vi "main.vi"() -> ()   [LabVIEW 2015]
doc: "Reading data from an ini file. Sorting using the array function. Writing sorted data to an ini file."
panel:
  out "errors when writing the ini file":errorcluster
  in  "Sorted and recorded file":path
  out "errors when reading the ini file":errorcluster
  in  "Source file":path
  in  "cluster structure":T1
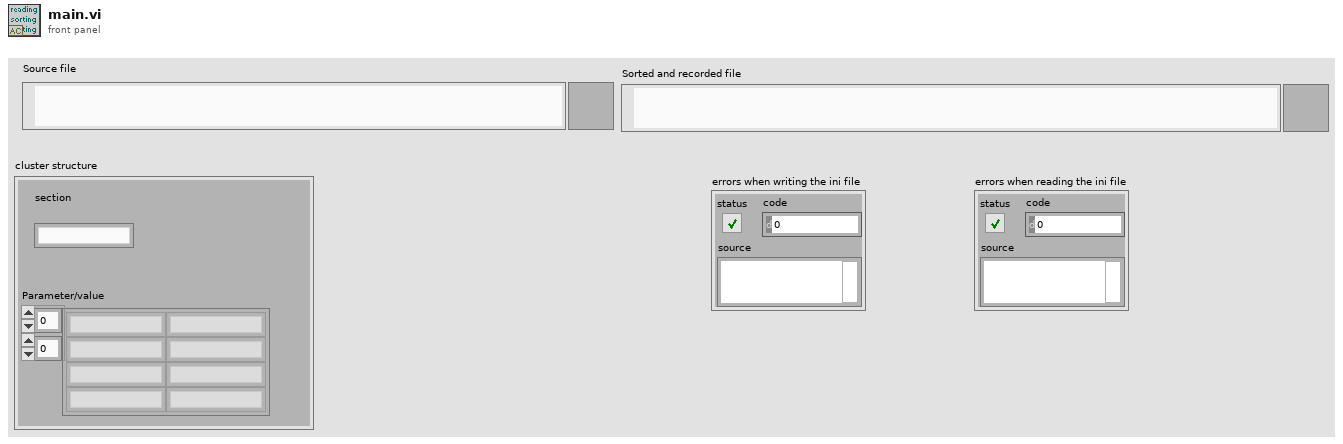
[diagram p1: front panel]
types:
  T1 = cluster{"section\n":string, "Parameter/value":string[][]}
  T2 = cluster{"Section":string, "Parameter/Value":string[][]}[]
  T3 = cluster{"Section":string, "Parametr/Value":string[][]}[]
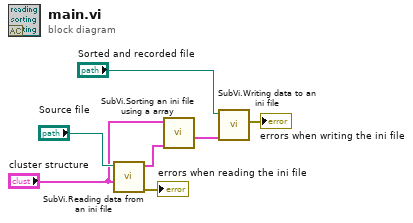
[diagram p0: block diagram]
diagram:
  n1 = call "SubVi.Reading data from an ini file.vi"("Data in the cluster"="cluster structure", "Source file"="Source file") -> ("error out"=→"errors when reading the ini file":errorcluster, "Array"=w5:T2)  [unwired: 4 in]
  n2 = call "SubVi.Sorting an ini file using a array.vi"("Input data"=w5, "Data in the cluster"="cluster structure") -> ("Output data"=w2:T3)  [unwired: 5 in]
  n3 = call "SubVi.Writing data to an ini file.vi"("Input data"=w2, "File with sorted\nand recorded data"="Sorted and recorded file") -> ("error"=→"errors when writing the ini file":errorcluster)  [unwired: 5 in]
